vi "Modify User.vi"(10 "User Type1":string, 11 "Path":path=path "E:/labview code/project user login/test1.txt") -> ()   [LabVIEW 2015]
panel:
  out "User Type":string
  in  "Password":string
  in  "User Name":string
  in  "Select User Name":u16(ring) items=["admin", "supervisor", "operator"]
  in  "MOdify":bool
  # "* Mandatory Field (Minimum length 4)"
  # "* Mandatory Field (Minimum length 4)"
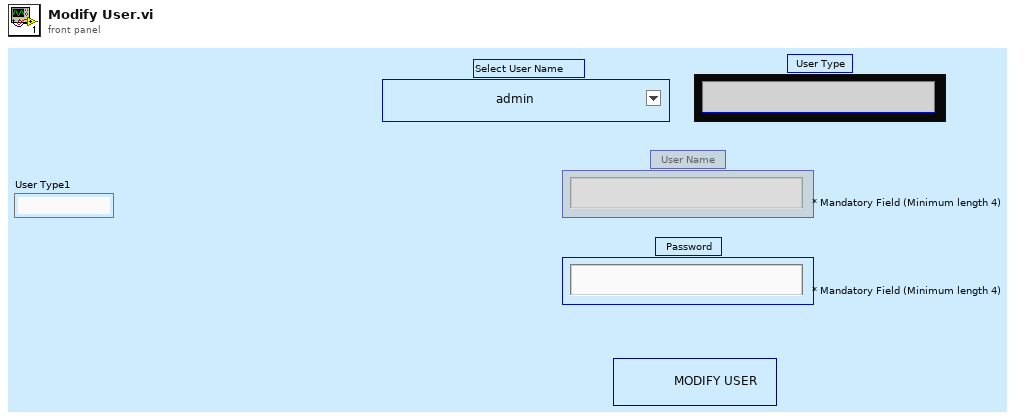
[diagram p1: front panel]
types:
  T1 = enum8{"Enabled", "Disabled", "Disabled and Grayed Out"}
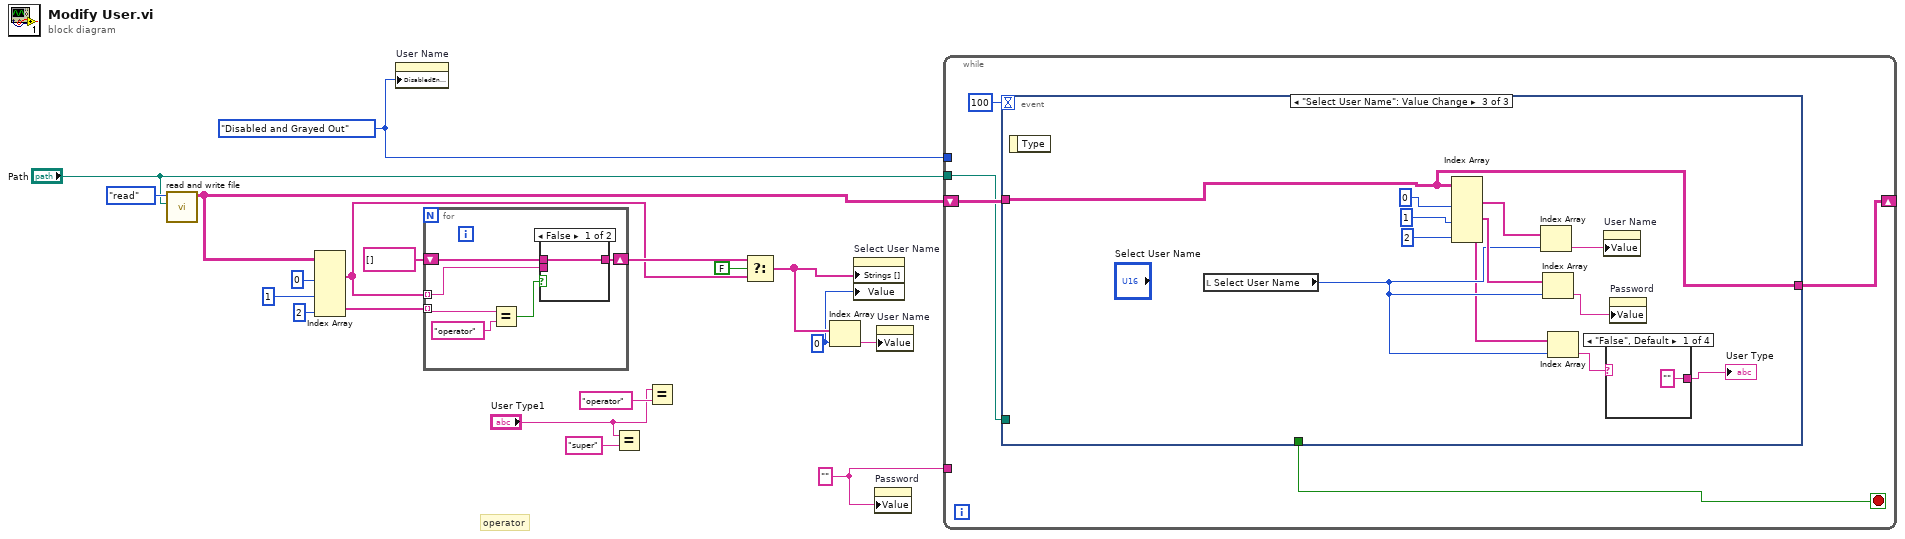
[diagram p0: block diagram]
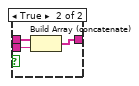
[diagram p2: hidden frame]
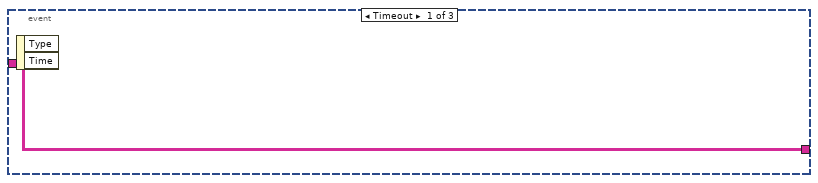
[diagram p3: hidden frame]
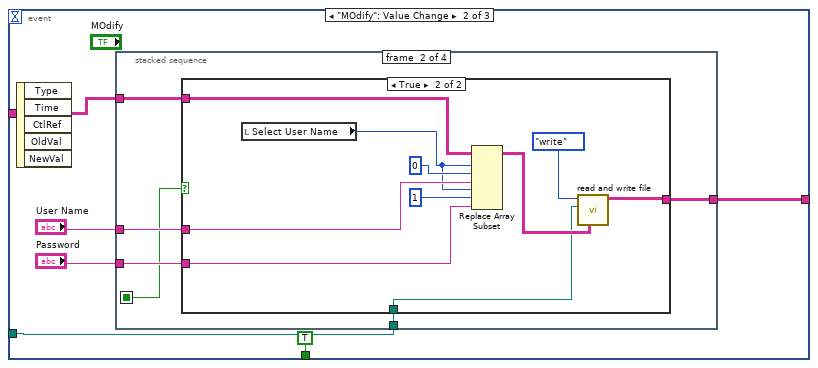
[diagram p4: hidden frame]
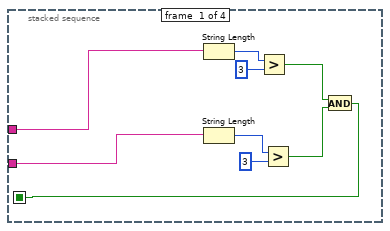
[diagram p5: hidden frame]
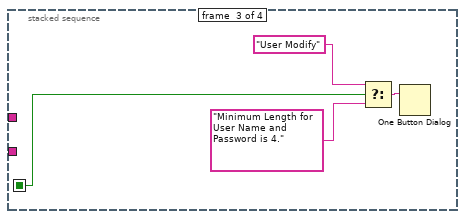
[diagram p7: hidden frame]
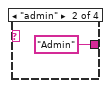
[diagram p9: hidden frame]
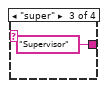
[diagram p10: hidden frame]
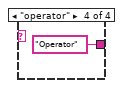
[diagram p11: hidden frame]
diagram:
  w1 = u16 0
  w19 = T1."Disabled and Grayed Out" ("Disabled")
  w7 = "" ("Password")
  # "operator"
  n1 = call "read and write file.vi"("Path"="Path", "Enum"=enum16{"write", "read"}."read") -> ("output data"=w14:string[][])  [unwired: 9 in]
  n2 = Index Array(array=w14, index (col) #1=0 ("index (row)"), index (col) #2=1 ("index (row)"), index (col) #3=2 ("index (col)")) -> (element #1=w8:string[], element #3=w10:string[])  [unwired: 3 in, 1 out]
  n3 = property on="User Name" class="Str"("DisabledEnum"=w19) -> ()  [unwired: 2 in, 2 out]
  n4 = for {
    tunnel: w10 -> [w25] mode=indexing
    tunnel: w8 -> [w22] mode=indexing
    shift-right: [w23] -> w11
    shift-left: string[] [] ("subarray") -> [w21]
    n5 = Equal?(x=w25, y="operator") -> (x = y?=w20:bool)
    n6 = case shown="False" w20 {
      tunnel: [w26 w29] -> w23
      tunnel: w22 -> [_ w28]
      tunnel: w21 -> [w26 w27]
      frame False {
      }
      frame True {
        n7 = Build Array (concatenate)(w27, w28) -> (w29:string[])
      }
    }
  }
  n8 = Equal?(x="User Type1", y="super") -> ()  [unwired: 1 out]
  n9 = Equal?(x="User Type1", y="operator") -> ()  [unwired: 1 out]
  n10 = Select(t=w11, s=FALSE, f=w8) -> (s? t:f=w6:string[])
  n11 = Index Array(array=w6, index=w1) -> (element=w5:string)
  n12 = property on="Select User Name" class="Ring (strict)"("Strings []"=w6, "Value"=w1) -> ()  [unwired: 2 in, 2 out]
  n13 = property on="Password" class="Str"("Value"=w7) -> ()  [unwired: 2 in, 2 out]
  n14 = property on="User Name" class="Str"("Value"=w5) -> ()  [unwired: 2 in, 2 out]
  n15 = while {
    tunnel: "Path" -> [w32]
    tunnel: w19 -> [_]
    tunnel: w7 -> [_]
    shift-right: [w31] -> _
    shift-left: w14 -> [w33]
    stop <- w34 stop-if-true
    n16 = event shown="[2] \"Select User Name\": Value Change" {
      selector: _ -> [_ _ _]
      dyn-events: _ -> [_ _ _]
      timeout: 100 -> [_ _ _]
      tunnel: w33 -> [w35 w41 w74]
      tunnel: [_ TRUE ("Exit 2") _] -> w34
      tunnel: w32 -> [_ w40 _]
      tunnel: [w35 w37 w74] -> w31
      event Timeout {
        n17 = event-data() -> ()  [unwired: 1 in, 2 out]
      }
      event "MOdify": Value Change {
        n18 = event-data() -> ()  [unwired: 1 in, 5 out]
        n19 = stacked-sequence {
          seq-local: [w42 _ _ _] -> [_ w52 w71 _]
          tunnel: w41 -> [_ w56 _ _]
          tunnel: w40 -> [_ w55 _ _]
          tunnel: "User Name" -> [w50 w54 _ _]
          tunnel: "Password" -> [w49 w53 _ _]
          tunnel: [_ w51 _ _] -> w37
          frame #0 {
            n20 = String Length(string=w50) -> (length=w48:i32)
            n21 = String Length(string=w49) -> (length=w45:i32)
            n22 = Greater?(x=w48, y=3) -> (0:w44:bool)
            n23 = Greater?(x=w45, y=3) -> (0:w43:bool)
            n24 = And(x=w44, y=w43) -> (x .and. y?=w42:bool)
          }
          frame #1 {
            n25 = case shown="True" w52 {
              tunnel: w56 -> [w57 w67]
              tunnel: w55 -> [_ w64]
              tunnel: w54 -> [_ w61]
              tunnel: w53 -> [_ w60]
              tunnel: [w57 w63] -> w51
              frame False {
              }
              frame True {
                n26 = local read "Select User Name"() -> (w59:u16)
                n27 = Replace Array Subset(array=w67, new element #1=w61, index (row) #1=w59, index (col) #1=0 ("disabled index (col)"), new element #2=w60, index (row) #2=w59, index (col) #2=1 ("disabled index (col)")) -> (w66:string[][])
                n28 = call "read and write file.vi"("data to write"=w66, "Path"=w64, "Enum"=enum16{"write", "read"}."write") -> ("output data"=w63:string[][])  [unwired: 8 in]
              }
            }
          }
          frame #2 {
            n29 = Select(t="User Modify" ("message"), s=w71, f="Minimum Length for User Name and Password is 4.") -> (s? t:f=w68:string)
            n30 = One Button Dialog(message=w68) -> ()  [unwired: 1 in, 1 out]
          }
          frame #3 {
          }
        }
      }
      event "Select User Name": Value Change {
        n31 = event-data() -> ()  [unwired: 1 in, 1 out]
        n32 = local read "Select User Name"() -> (w77:u16)
        n33 = Index Array(array=w74, index (col) #1=0 ("index (row)"), index (col) #2=1 ("index (row)"), index (col) #3=2 ("index (row)")) -> (element #1=w79:string[], element #2=w78:string[], element #3=w75:string[])  [unwired: 3 in]
        n34 = Index Array(array=w79, index=w77) -> (element=w80:string)
        n35 = Index Array(array=w78, index=w77) -> (element=w81:string)
        n36 = Index Array(array=w75, index=w77) -> (element=w73:string)
        n37 = property on="User Name" class="Str"("Value"=w80) -> ()  [unwired: 2 in, 2 out]
        n38 = case shown="\"False\", Default" w73 {
          tunnel: ["" ("y") "Admin" ("y") "Supervisor" ("y") "Operator" ("y")] -> w72
          frame "False", Default {
          }
          frame "admin" {
          }
          frame "super" {
          }
          frame "operator" {
          }
        }
        "User Type" <- w72
        n39 = property on="Password" class="Str"("Value"=w81) -> ()  [unwired: 2 in, 2 out]
      }
    }
  }
